vi "Read Drive Encoders.vi"(13 "Input Array":dbl[](array[numeric])) -> (2 "Appended Array":dbl[](array[numeric]), 6 "Drive Encoder BR":dbl, 8 "Drive Encoder BL":dbl, 10 "Drive Encoder FR":dbl, 15 "Drive Encoder FL":dbl)   [LabVIEW 2014]
uses:
  Begin/Global RefNums.vi
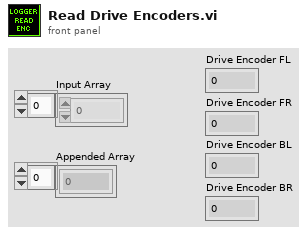
[diagram p1: front panel]
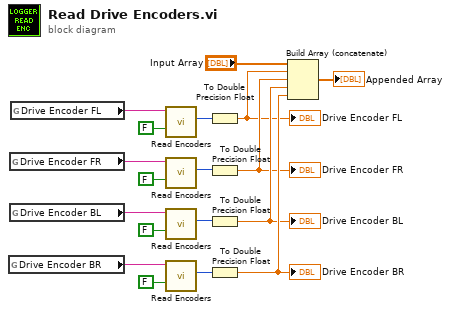
[diagram p0: block diagram]
diagram:
  n1 = global read "Global RefNums.vi" "Drive Encoder BR"() -> (w10:string)
  n2 = global read "Global RefNums.vi" "Drive Encoder FR"() -> (w12:string)
  n3 = global read "Global RefNums.vi" "Drive Encoder BL"() -> (w7:string)
  n4 = global read "Global RefNums.vi" "Drive Encoder FL"() -> (w11:string)
  n5 = call "Read Encoders.vi"("Reset Encoders"=FALSE, "Encoder"=w11) -> ("Counts"=w17:i32)  [unwired: 9 in]
  n6 = call "Read Encoders.vi"("Reset Encoders"=FALSE, "Encoder"=w12) -> ("Counts"=w16:i32)  [unwired: 9 in]
  n7 = call "Read Encoders.vi"("Reset Encoders"=FALSE, "Encoder"=w7) -> ("Counts"=w15:i32)  [unwired: 9 in]
  n8 = call "Read Encoders.vi"("Reset Encoders"=FALSE, "Encoder"=w10) -> ("Counts"=w18:i32)  [unwired: 9 in]
  n9 = To Double Precision Float(number=w17) -> (double precision float=w1:dbl)
  "Drive Encoder FL" <- w1
  n10 = To Double Precision Float(number=w16) -> (double precision float=w2:dbl)
  "Drive Encoder FR" <- w2
  n11 = To Double Precision Float(number=w15) -> (double precision float=w3:dbl)
  "Drive Encoder BL" <- w3
  n12 = To Double Precision Float(number=w18) -> (double precision float=w4:dbl)
  "Drive Encoder BR" <- w4
  n13 = Build Array (concatenate)("Input Array", w1, w2, w3, w4) -> (→"Appended Array":dbl[])
